vi "WriteConfig.vi"(8 "error in (no error)":errorcluster, 10 "Config":variant, 11 "C37.118 Sim in":refnum<class "C37.118 Sim.lvclass">) -> (0 "error out":errorcluster, 3 "C37.118 Sim out":refnum<class "C37.118 Sim.lvclass">)   [LabVIEW 2014, in "SensorPlugins.lvlib" / "C37.118 Sim.lvclass"]
uses:
  C37.118 Sim.lvclass
  PmuBaseClass/PmuBase.lvclass
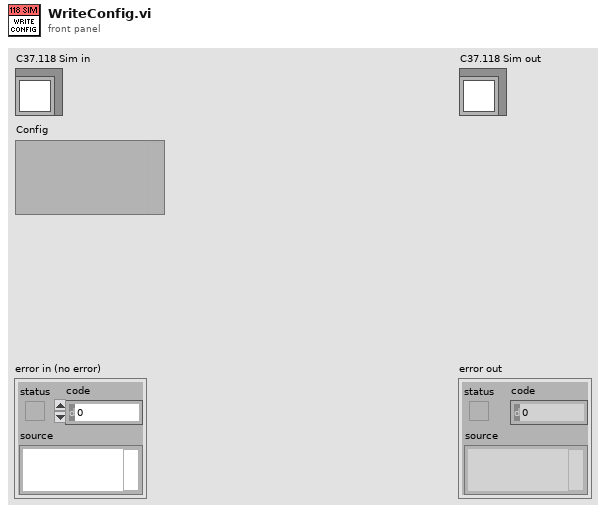
[diagram p1: front panel]
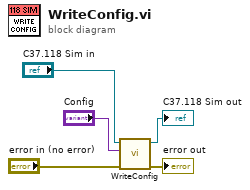
[diagram p0: block diagram]
diagram:
  n1 = call-parent "WriteConfig.vi"("error in (no error)"="error in (no error)", "Config"="Config", "PmuBase in"="C37.118 Sim in") -> ("error out"=→"error out":errorcluster, "PmuBase out"=→"C37.118 Sim out":refnum<class "C37.118 Sim.lvclass">)  [unwired: 7 in]
